vi "Convert Number of Seconds to Running Time.vi"(1 "Use Full Unit Names? (F)":bool, 2 "Number of seconds elapsed":dbl format="%#_10f") -> (0 "Running Time String":string)   [LabVIEW 2016, in "Error Manager.lvlib"]
doc: "This VI is suited to formatting the running time of long-running apps, that may run for days, or even months, or years at a time.\n\nConverts the number of seconds to a human-friendly \"Running Time\" string.\nExamples:\n0 seconds to \"0 s\"\n1 seconds to \"1 s\"\n59 seconds to \"59 s\"\n60 seconds to \"1 m 0 s\"\n61 seconds to \"1 m 1 s\"\n3600 seconds to \"1 h 0 m 0 s\"\n3601 seconds to \"1 h 0 m 1 s\"\n3661 seconds to \"1 h 1 m 1 s\"\n113684 seconds to \"1 day 7 h 34 m 44 s\"\n1113684 seconds to \"12 days 21 h 21 m 24 s\"\n111113684 seconds to \"1286 days 0 h 54 m 44 s\""
uses:
  Error Manager.lvlib
panel:
  # "Development\nControls or indicators that are useful for development or testing, but which are not outputs of the VI."
  # "Input\nInputs to the VI"
  # "Output\nOutputs of the VI"
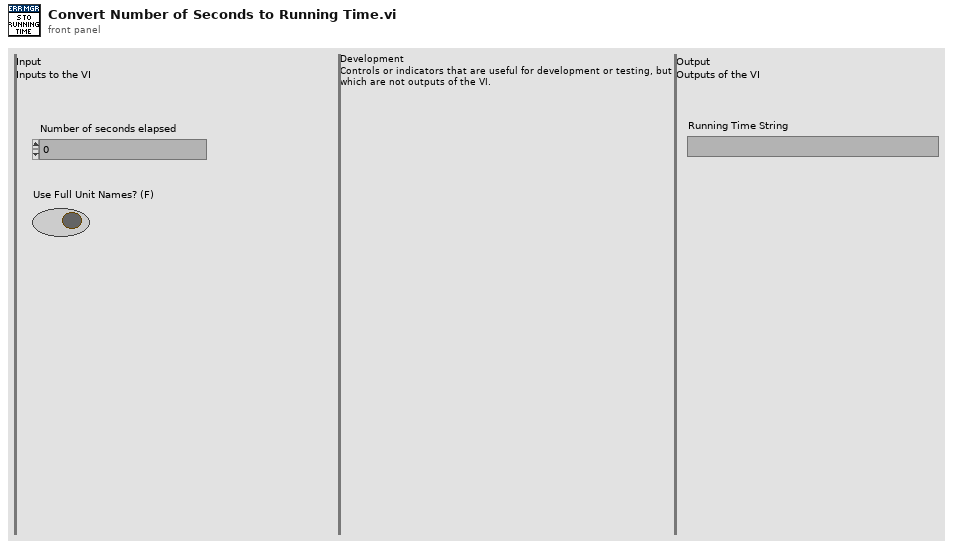
[diagram p1: front panel]
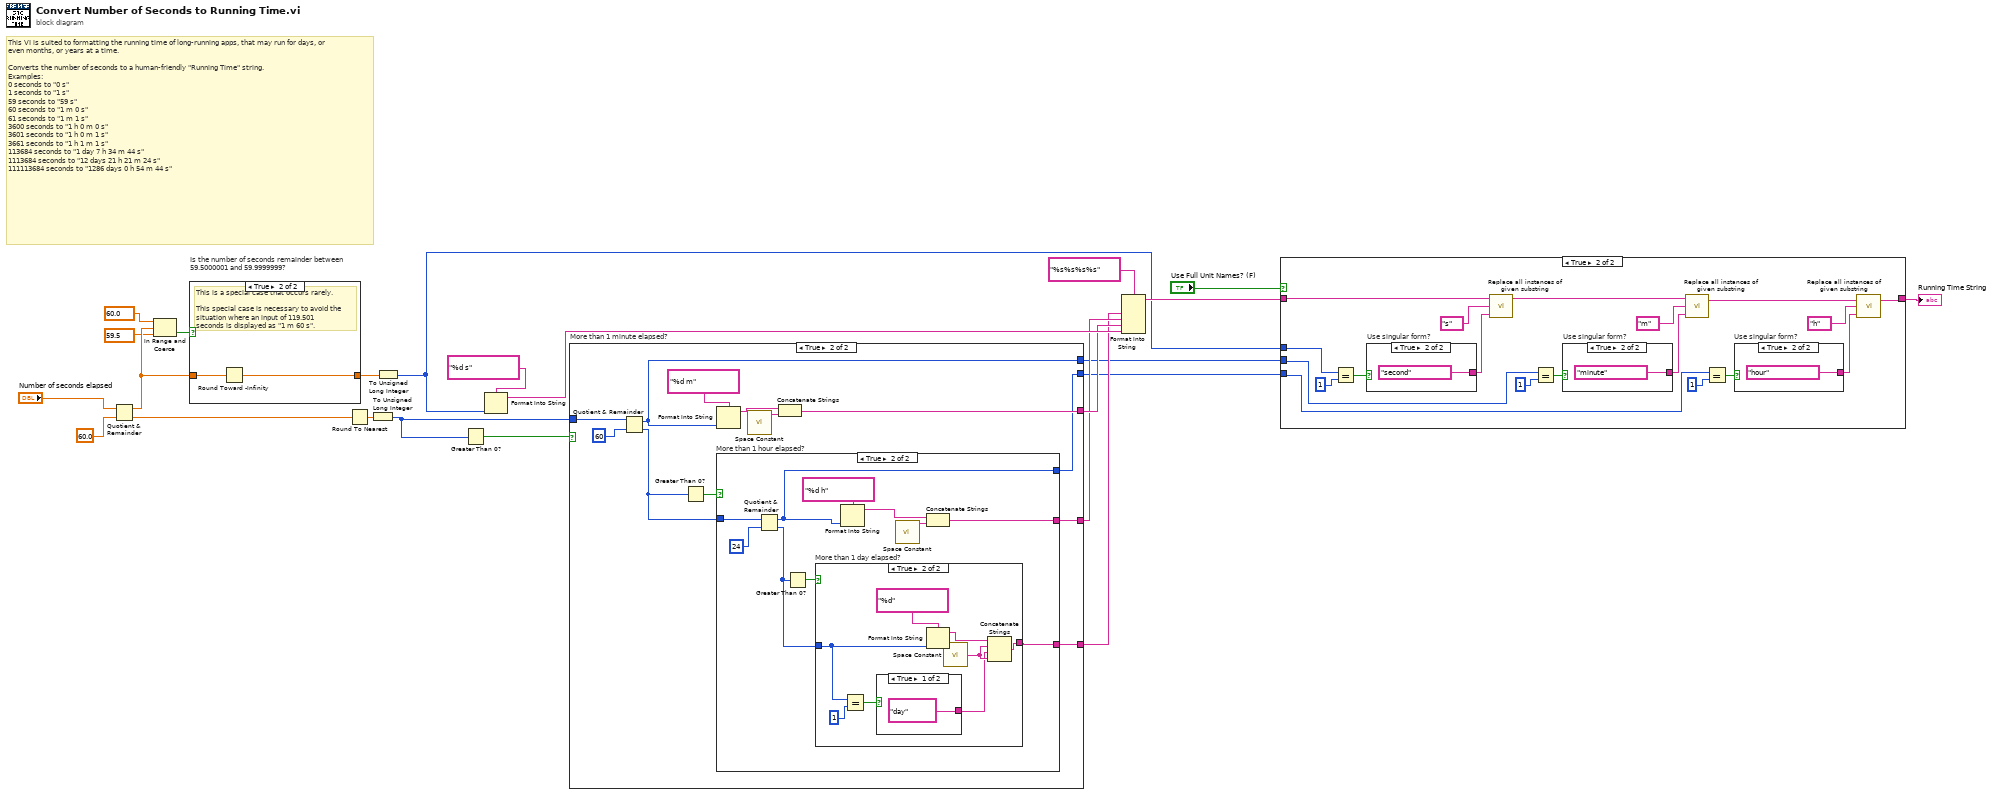
[diagram p0: block diagram]
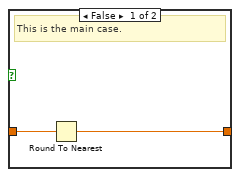
[diagram p2: hidden frame]
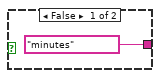
[diagram p4: hidden frame]
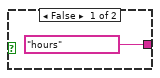
[diagram p5: hidden frame]
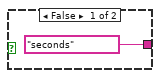
[diagram p6: hidden frame]
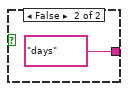
[diagram p10: hidden frame]
diagram:
  # "This VI is suited to formatting the running time of long-running apps, that may run for days, or even months, or years at a time.\n\nConverts the number of seconds to a human-friendly \"Running Time\" string.\nExamples:\n0 seconds to \"0 s\"\n1 seconds to \"1 s\"\n59 seconds to \"59 s\"\n60 seconds to \"1 m 0 s\"\n61 seconds to \"1 m 1 s\"\n3600 seconds to \"1 h 0 m 0 s\"\n3601 seconds to \"1 h 0 m 1 s\"\n3661 seconds to \"1 h 1 m 1 s\"\n113684 seconds to \"1 day 7 h 34 m 44 s\"\n1113684 seconds to \"12 days 21 h 21 m 24 s\"\n111113684 seconds to \"1286 days 0 h 54 m 44 s\""
  n1 = Quotient & Remainder(x="Number of seconds elapsed", y=60.0) -> (x-y*floor(x/y)=w4:dbl, floor(x/y)=w17:dbl)
  n2 = In Range and Coerce(upper limit=60.0 ("y"), x=w4, lower limit=59.5 ("y")) -> (In Range?=w1:bool)  [unwired: 1 out]
  n3 = case "Is the number of seconds remainder between 59.5000001 and 59.9999999?" shown="True" w1 {
    tunnel: [w25 w26] -> w6
    tunnel: w4 -> [w24 w27]
    frame False {
      # "This is the main case."
      n4 = Round To Nearest(number=w24) -> (nearest integer value=w25:dbl)
    }
    frame True {
      # "This is a special case that occurs rarely.\n\nThis special case is necessary to avoid the situation where an input of 119.501 seconds is displayed as \"1 m 60 s\"."
      n5 = Round Toward -Infinity(1:w27) -> (0:w26:dbl)
    }
  }
  n6 = Round To Nearest(number=w17) -> (nearest integer value=w15:dbl)
  n7 = To Unsigned Long Integer(number=w15) -> (unsigned 32bit integer=w14:u32)
  n8 = To Unsigned Long Integer(number=w6) -> (unsigned 32bit integer=w5:u32)
  n9 = Greater Than 0?(x=w14) -> (x > 0?=w21:bool)
  n10 = Format Into String(format string="%d s", w5) -> (resulting string=w18:string)  [unwired: 2 in, 1 out]
  n11 = case "More than 1 minute elapsed?" shown="True" w21 {
    tunnel: w14 -> [_ w38]
    tunnel: [_ w34] -> w16
    tunnel: [_ w32] -> w13
    tunnel: [_ w30] -> w12
    tunnel: [_ w29] -> w8
    tunnel: [_ w28] -> w7
    frame False {
    }
    frame True {
      n12 = Quotient & Remainder(x=w38, y=u32 60) -> (x-y*floor(x/y)=w29:u32, floor(x/y)=w31:u32)
      n13 = Greater Than 0?(x=w31) -> (x > 0?=w33:bool)
      n14 = Format Into String(format string="%d m", w29) -> (resulting string=w36:string)  [unwired: 2 in, 1 out]
      n15 = case "More than 1 hour elapsed?" shown="True" w33 {
        tunnel: w31 -> [_ w45]
        tunnel: [_ w46] -> w32
        tunnel: [_ w41] -> w30
        tunnel: [_ w40] -> w28
        frame False {
        }
        frame True {
          n16 = Quotient & Remainder(x=w45, y=u32 24) -> (x-y*floor(x/y)=w40:u32, floor(x/y)=w42:u32)
          n17 = Greater Than 0?(x=w42) -> (x > 0?=w43:bool)
          n18 = case "More than 1 day elapsed?" shown="True" w43 {
            tunnel: [_ w55] -> w41
            tunnel: w42 -> [_ w54]
            frame False {
            }
            frame True {
              n19 = Equal?(x=w54, y=u32 1) -> (x = y?=w51:bool)
              n20 = case shown="True" w51 {
                tunnel: ["day" "days"] -> w50
                frame True {
                }
                frame False {
                }
              }
              n21 = Format Into String(format string="%d", w54) -> (resulting string=w56:string)  [unwired: 2 in, 1 out]
              n22 = call <vilib>:"Space Constant.vi"() -> ("String"=w53:string)
              n23 = Concatenate Strings(w56, w53, w50, w53) -> (w55:string)
            }
          }
          n24 = Format Into String(format string="%d h", w40) -> (resulting string=w47:string)  [unwired: 2 in, 1 out]
          n25 = call <vilib>:"Space Constant.vi"() -> ("String"=w48:string)
          n26 = Concatenate Strings(w47, w48) -> (w46:string)
        }
      }
      n27 = call <vilib>:"Space Constant.vi"() -> ("String"=w35:string)
      n28 = Concatenate Strings(w36, w35) -> (w34:string)
    }
  }
  n29 = Format Into String(format string="%s%s%s%s", w12, w13, w16, w18) -> (resulting string=w11:string)  [unwired: 2 in, 1 out]
  n30 = case shown="True" "Use Full Unit Names? (F)" {
    tunnel: w11 -> [w60 w70]
    tunnel: [w60 w64] -> w9
    tunnel: w8 -> [_ w63]
    tunnel: w7 -> [_ w61]
    tunnel: w5 -> [_ w75]
    frame False {
    }
    frame True {
      n31 = Equal?(x=w75, y=u32 1) -> (x = y?=w76:bool)
      n32 = case "Use singular form?" shown="True" w76 {
        tunnel: ["seconds" ("Substring 1 (find and replace this)") "second" ("Substring 1 (find and replace this)")] -> w78
        frame False {
        }
        frame True {
        }
      }
      n33 = call "Replace all instances of given substring.vi"("Substring 2 (replace with this)"=w78, "Substring 1 (find and replace this)"="s", "String In"=w70) -> ("String Out (all instances of substring 1 replaced with substring 2)"=w66:string)  [unwired: 1 out]
      n34 = Equal?(x=w63, y=u32 1) -> (x = y?=w62:bool)
      n35 = case "Use singular form?" shown="True" w62 {
        tunnel: ["minutes" ("Substring 1 (find and replace this)") "minute" ("Substring 1 (find and replace this)")] -> w69
        frame False {
        }
        frame True {
        }
      }
      n36 = call "Replace all instances of given substring.vi"("Substring 2 (replace with this)"=w69, "Substring 1 (find and replace this)"="m", "String In"=w66) -> ("String Out (all instances of substring 1 replaced with substring 2)"=w65:string)  [unwired: 1 out]
      n37 = Equal?(x=w61, y=u32 1) -> (x = y?=w74:bool)
      n38 = case "Use singular form?" shown="True" w74 {
        tunnel: ["hours" ("Substring 1 (find and replace this)") "hour" ("Substring 1 (find and replace this)")] -> w73
        frame False {
        }
        frame True {
        }
      }
      n39 = call "Replace all instances of given substring.vi"("Substring 2 (replace with this)"=w73, "Substring 1 (find and replace this)"="h", "String In"=w65) -> ("String Out (all instances of substring 1 replaced with substring 2)"=w64:string)  [unwired: 1 out]
    }
  }
  "Running Time String" <- w9
